vi "SLL Is Exe.vi"(8 "error in (no error)":errorcluster) -> (0 "error out":errorcluster, 3 "Is Exe?":bool)   [LabVIEW 2013]
doc: "Finds the application kind. Gives out TRUE if the appication is Executable.\n\nCopyright © 2006, Soliton Technologies. All rights reserved."
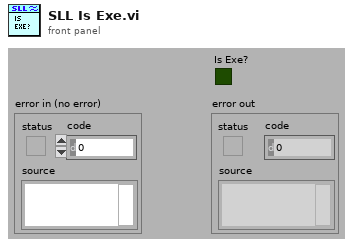
[diagram p1: front panel]
types:
  T1 = enum32{"invalid app kind", "Development System", "Run Time System", "Student Edition", "Embedded LabVIEW"}
  T2 = enum32{"invalid app kind", "Development System", "Run Time System", "Student Edition", "Embedded LabVIEW", "Evaluation", "Custom"}
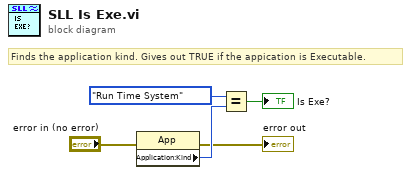
[diagram p0: block diagram]
diagram:
  # "Finds the application kind. Gives out TRUE if the appication is Executable."
  n1 = property class="App"(error in="error in (no error)") -> (error out=→"error out":errorcluster, "Application:Kind"=w5:T2)  [unwired: 1 in, 1 out]
  n2 = Equal?(x=T1."Run Time System" ("Application:Kind"), y=w5) -> (x = y?=→"Is Exe?":bool)
